vi "Get Param.vi"(0 "paramID":i32, 1 "error in (no error)":errorcluster) -> (2 "function return":i32, 3 "param out":dbl, 4 "error out":errorcluster)   [LabVIEW 2014, in "MPH16.lvlib"]
doc: "long GetParam(const long paramID, double &param);"
uses:
  MPH16.lvlib
  ThorPinholeStepper.dll
panel:
  in  "param":dbl
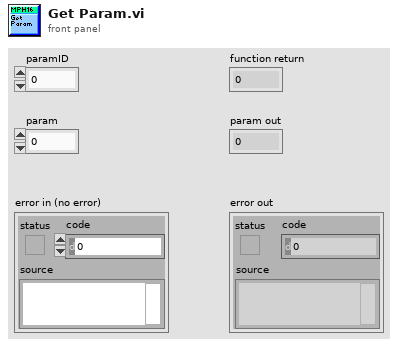
[diagram p1: front panel]
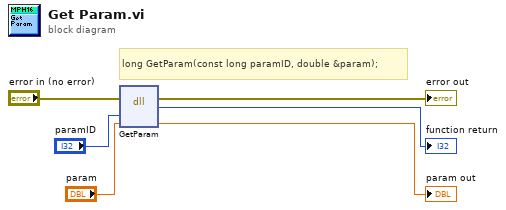
[diagram p0: block diagram]
diagram:
  # "long GetParam(const long paramID, double &param);"
  n1 = dll-call lib="C:/TIS_CalebVS2012/TIS_Development/Hardware/SDKs/MPH16_SDK/LabVIEW/inc/ThorPinholeStepper.*" fn="GetParam"(error in="error in (no error)", "paramID"="paramID", "param"="param") -> (error out=→"error out":errorcluster, →"function return":i32, "param"=→"param out":dbl)  [unwired: 3 in, 1 out]
